vi "ArrayBytes to string.vi"(0 "Array Bytes":u8[](array[numeric]), 1 "Sigle length+2":u16, 2 "Char/Str":bool, 3 "item":u16) -> (5 "String":string[](array[string]))   [LabVIEW 2014, in "Simatic S7.lvlib"]
uses:
  Simatic S7.lvlib
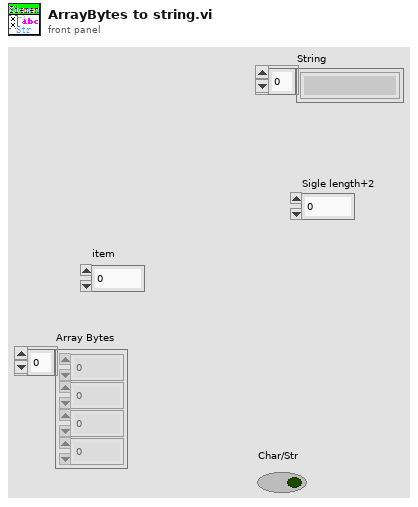
[diagram p1: front panel]
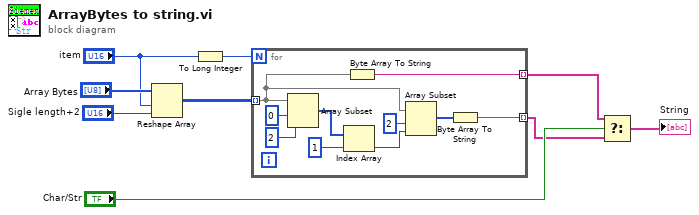
[diagram p0: block diagram]
diagram:
  n1 = Reshape Array("Array Bytes", "item", "Sigle length+2") -> (w5:u8[][])
  n2 = To Long Integer(number="item") -> (32bit integer=w9:i32)
  n3 = for {
    N: w9 -> [_]
    tunnel: w5 -> [w10] mode=indexing
    tunnel: [w13] -> w2 mode=indexing
    tunnel: [w11] -> w1 mode=indexing
    n4 = Array Subset(array=w10, index=0, length=2) -> (w12:u8[])
    n5 = Index Array(array=w12, index=1) -> (element=w15:u8)
    n6 = Byte Array To String(unsigned byte array=w10) -> (string=w11:string)
    n7 = Array Subset(array=w10, index=2, length=w15) -> (w14:u8[])
    n8 = Byte Array To String(unsigned byte array=w14) -> (string=w13:string)
  }
  n9 = Select(t=w1, s="Char/Str", f=w2) -> (s? t:f=→"String":string[])
